vi "ief_abort_auto.vi"(2 "error in (no error)":errorcluster, 3 "Tagprefix in":refnum<k21>) -> (0 "error out (no error)":errorcluster, 1 "Tagprefix out":refnum<k21>)   [LabVIEW 2015, in "IEF Werner.lvlib"]
doc: "The VI stops positioning and aborts the automatic mode. The PA control state is switched to basic mode."
uses:
  IEF Werner.lvlib
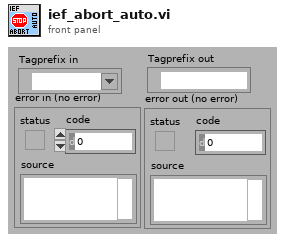
[diagram p1: front panel]
types:
  T1 = typedef "Semaphore RefNum" = refnum<k1>
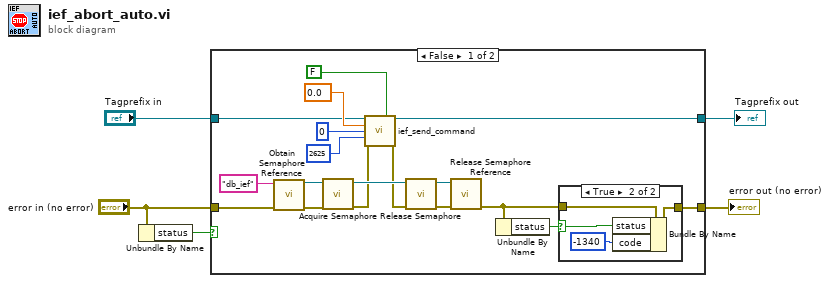
[diagram p0: block diagram]
diagram:
  n1 = Unbundle By Name("error in (no error)") -> ("status"=w3:bool)
  n2 = case shown="False" w3 {
    tunnel: "error in (no error)" -> [w14 w30]
    tunnel: [w21 w30] -> w5
    tunnel: "Tagprefix in" -> [w7 w29]
    tunnel: [w6 w29] -> w1
    frame False {
      n3 = call <vilib>:"Obtain Semaphore Reference.vi"("error in (no error)"=w14, "name (unnamed)"="db_ief") -> ("error out"=w18:errorcluster, "semaphore"=w19:T1)  [unwired: 3 in, 1 out]
      n4 = call <vilib>:"Acquire Semaphore.vi"("error in (no error)"=w18, "semaphore"=w19) -> ("error out"=w13:errorcluster, "semaphore out"=w17:T1)  [unwired: 3 in, 1 out]
      n5 = call "ief_send_command.vi"("Tagprefix in"=w7, "Command datum of type real"=FALSE, "Command datum"=sgl 0.0, "Command parameter"=u16 0, "Command code"=u16 2625, "error in (no error)"=w13) -> ("Tagprefix out"=w6:refnum<k21>, "error out (no error)"=w8:errorcluster)  [unwired: 4 in, 4 out]
      n6 = call <vilib>:"Release Semaphore.vi"("error in (no error)"=w8, "semaphore"=w17) -> ("error out"=w16:errorcluster, "semaphore out"=w15:T1)  [unwired: 4 in]
      n7 = call <vilib>:"Release Semaphore Reference.vi"("error in (no error)"=w16, "semaphore"=w15) -> ("error out"=w12:errorcluster)  [unwired: 8 in, 1 out]
      n8 = Unbundle By Name(w12) -> ("status"=w9:bool)
      n9 = case shown="True" w9 {
        selector: w9 -> [_ w25]
        tunnel: [w24 w27] -> w21
        tunnel: w12 -> [w24 w28]
        frame False {
        }
        frame True {
          n10 = Bundle By Name(cluster=w28, "status"=w25, "code"=-1340) -> (w27:errorcluster)
        }
      }
    }
    frame True {
    }
  }
  "error out (no error)" <- w5
  "Tagprefix out" <- w1
